vi "Normalize Position.vi"(7 "Size":i32, 10 "Col In":i32, 11 "Row In":i32) -> (2 "Col":i32, 3 "Row":i32)   [LabVIEW 2020, in "SquareBattle.lvlib"]
doc: "Ensures a position is wrapped around the edges of the game field properly. E.g. if a position is off the top edge of the field, it will wrap around the bottom."
uses:
  SquareBattle.lvlib
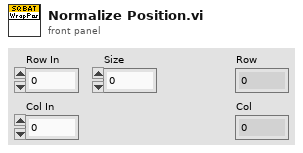
[diagram p1: front panel]
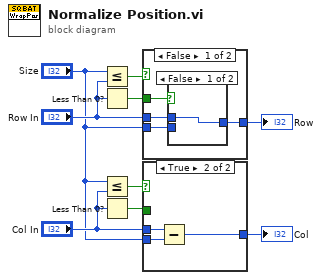
[diagram p0: block diagram]
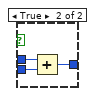
[diagram p3: hidden frame]
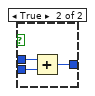
[diagram p4: hidden frame]
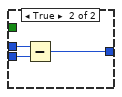
[diagram p5: hidden frame]
diagram:
  n1 = Less Or Equal?(x="Size", y="Row In") -> (x <= y?=w9:bool)
  n2 = Less Than 0?(x="Row In") -> (x < 0?=w8:bool)
  n3 = Less Or Equal?(x="Size", y="Col In") -> (x <= y?=w7:bool)
  n4 = Less Than 0?(x="Col In") -> (x < 0?=w6:bool)
  n5 = case shown="False" w9 {
    tunnel: w8 -> [w13 _]
    tunnel: "Row In" -> [w12 w20]
    tunnel: "Size" -> [w11 w19]
    tunnel: [w10 w18] -> w1
    frame False {
      n6 = case shown="False" w13 {
        tunnel: w12 -> [w14 w17]
        tunnel: w11 -> [_ w16]
        tunnel: [w14 w15] -> w10
        frame False {
        }
        frame True {
          n7 = Add(x=w17, y=w16) -> (x+y=w15:i32)
        }
      }
    }
    frame True {
      n8 = Subtract(x=w20, y=w19) -> (x-y=w18:i32)
    }
  }
  "Row" <- w1
  n9 = case shown="True" w7 {
    tunnel: w6 -> [w24 _]
    tunnel: "Col In" -> [w23 w31]
    tunnel: "Size" -> [w22 w30]
    tunnel: [w21 w29] -> w2
    frame False {
      n10 = case shown="False" w24 {
        tunnel: w23 -> [w25 w28]
        tunnel: w22 -> [_ w27]
        tunnel: [w25 w26] -> w21
        frame False {
        }
        frame True {
          n11 = Add(x=w28, y=w27) -> (x+y=w26:i32)
        }
      }
    }
    frame True {
      n12 = Subtract(x=w31, y=w30) -> (x-y=w29:i32)
    }
  }
  "Col" <- w2
